vi "OP40 Indicators.vi"(8 "error in (no error)":errorcluster, 10 "Array":refnum<vi>[](array[refnum]), 11 "OUTPUT INDICATOR in":T1) -> (0 "error out":errorcluster, 3 "OUTPUT INDICATOR out":T1)   [LabVIEW 2017]
uses:
  f441d0c3-00bd-40e1-bd83-0ce583e46ada.vi
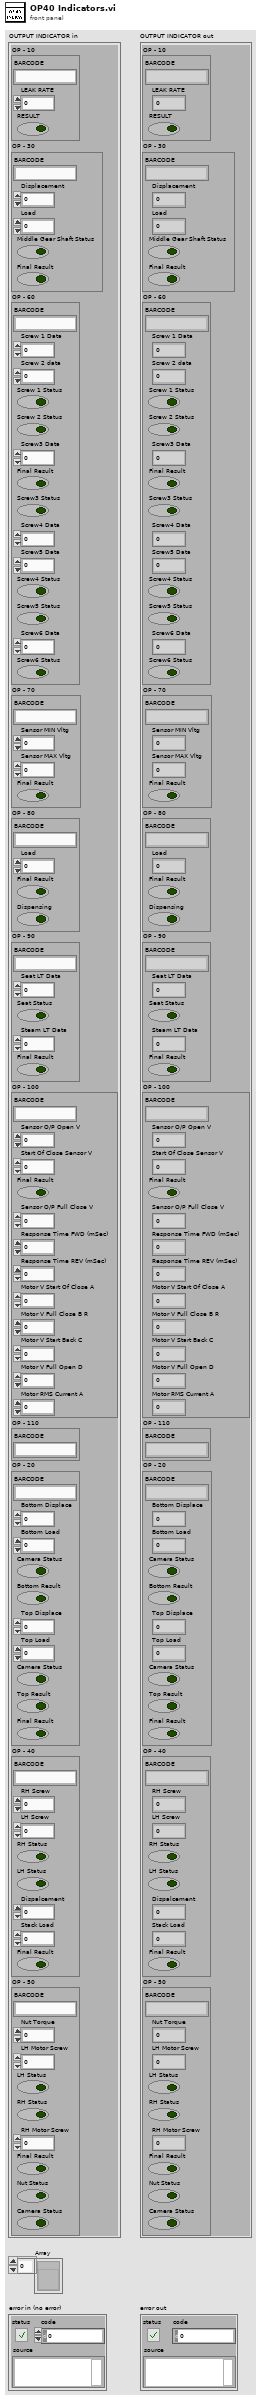
[diagram p1: front panel]
types:
  T1 = cluster{"OP - 10":cluster{"BARCODE":string, "LEAK RATE":dbl, "RESULT":bool}, "OP - 30":cluster{"BARCODE":string, "Displacement":dbl, "Load":dbl, "Middle Gear Shaft Status":bool, "Final Result":bool}, "OP - 60":cluster{"BARCODE":string, "Screw 1 Data":dbl, "Screw 2 data":dbl, "Screw 1 Status":bool, "Screw 2 Status":bool, "Screw3 Data":dbl, "Final Result":bool, "Screw3 Status":bool, "Screw4 Data":dbl, "Screw5 Data":dbl, "Screw4 Status":bool, "Screw5 Status":bool, "Screw6 Data":dbl, "Screw6 Status":bool}, "OP - 70":cluster{"BARCODE":string, "Sensor MIN Vltg":dbl, "Sensor MAX Vltg":dbl, "Final Result":bool}, "OP - 80":cluster{"BARCODE":string, "Load":dbl, "Final Result":bool, "Dispensing":bool}, "OP - 90":cluster{"BARCODE":string, "Seat LT Data":dbl, "Seat Status":bool, "Steam LT Data":dbl, "Final Result":bool}, "OP - 100":cluster{"BARCODE":string, "Sensor O/P Open V":dbl, "Start Of Close Sensor V":dbl, "Final Result":bool, "Sensor O/P Full Close V":dbl, "Response Time FWD (mSec)":dbl, "Response Time REV (mSec)":dbl, "Motor V Start Of Close A":dbl, "Motor V Full Close B R":dbl, "Motor V Start Back C":dbl, "Motor V Full Open D":dbl, "Motor RMS Current A":dbl}, "OP - 110":cluster{"BARCODE":string}, "OP - 20":cluster{"BARCODE":string, "Bottom Displace":dbl, "Bottom Load":dbl, "Camera Status":bool, "Bottom Result":bool, "Top Displace":dbl, "Top Load ":dbl, "Camera Status":bool, "Top Result":bool, "Final Result":bool}, "OP - 40":cluster{"BARCODE":string, "RH Screw":dbl, "LH Screw ":dbl, "RH Status":bool, "LH Status":bool, "Dispalcement ":dbl, "Stack Load ":dbl, "Final Result":bool}, "OP - 50":cluster{"BARCODE":string, "Nut Torque":dbl, "LH Motor Screw":dbl, "LH Status":bool, "RH Status":bool, "RH Motor Screw":dbl, "Final Result":bool, "Nut Status":bool, "Camera Status":bool}}
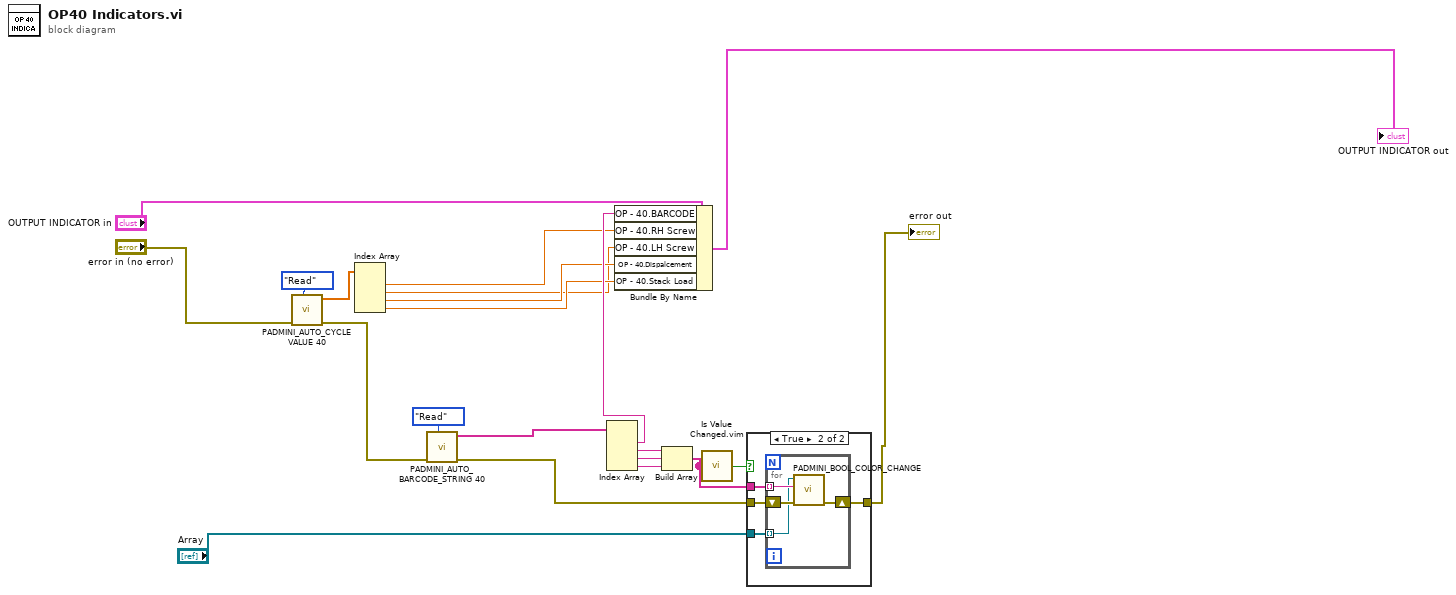
[diagram p0: block diagram]
diagram:
  n1 = call "PADMINI_AUTO_CYCLE VALUE 40.vi"("Enum"=enum16{"Read", "Write"}."Read", "error in (no error)"="error in (no error)") -> ("error out"=w10:errorcluster, "Input 2"=w3:sgl[])  [unwired: 8 in]
  n2 = Index Array(array=w3) -> (element #1=w5:sgl, element #2=w6:sgl, element #3=w7:sgl, element #4=w8:sgl)  [unwired: 4 in]
  n3 = call "PADMINI_AUTO_BARCODE_STRING 40.vi"("Enum"=enum16{"Read", "Write"}."Read", "error in (no error)"=w10) -> ("error out"=w17:errorcluster, "Input 2"=w15:string[])  [unwired: 8 in]
  n4 = Index Array(array=w15) -> (element #1=w16:string, element #2=w12:string, element #3=w13:string, element #4=w19:string)  [unwired: 4 in]
  n5 = Bundle By Name(cluster="OUTPUT INDICATOR in", "OP - 40.BARCODE"=w16, "OP - 40.RH Screw"=w5, "OP - 40.LH Screw"=w6, "OP - 40.Dispalcement"=w7, "OP - 40.Stack Load"=w8) -> (→"OUTPUT INDICATOR out":T1)
  n6 = Build Array(w12, w13, w19) -> (w14:string[])
  n7 = call "Is Value Changed.vim"("value"=w14) -> ("changed or first call?"=w11:bool)
  n8 = case shown="True" w11 {
    tunnel: [w22 w26] -> w20
    tunnel: w14 -> [_ w25]
    tunnel: w17 -> [w22 w24]
    tunnel: "Array" -> [_ w23]
    frame False {
    }
    frame True {
      n9 = for {
        tunnel: w25 -> [w29] mode=indexing
        shift-right: [w30] -> w26
        shift-left: w24 -> [w28]
        tunnel: w23 -> [w27] mode=indexing
        n10 = call "PADMINI_BOOL_COLOR_CHANGE.vi"("error in (no error)"=w28, "Input Result"=w29, "Boolean in"=w27) -> ("error out"=w30:errorcluster)  [unwired: 8 in]
      }
    }
  }
  "error out" <- w20
